vi "read_node_object_dictionary.vi"(0 "node":u8, 5 "index":u16, 7 "subind":u8, 9 "upd":u8, 11 "num":u64) -> (4 "return":i16, 6 "upd":u8, 8 "num":u64)   [LabVIEW 2011]
uses:
  canopen_dll_master.dll
panel:
  in  "num":cluster{"num":u64}
  in  "upd":cluster{"upd":u8}
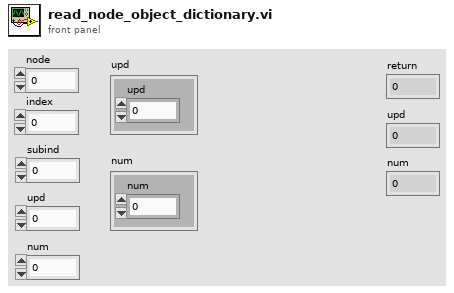
[diagram p1: front panel]
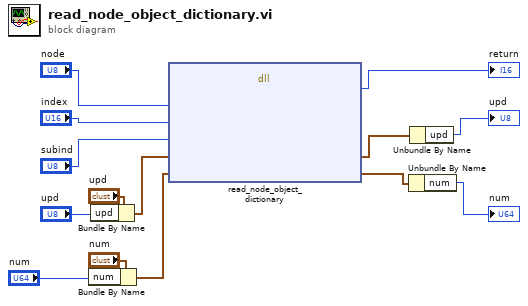
[diagram p0: block diagram]
diagram:
  n1 = Bundle By Name(cluster="num", "num"="num") -> (w3:cluster{"num":u64})
  n2 = Bundle By Name(cluster="upd", "upd"="upd") -> (w9:cluster{"upd":u8})
  n3 = dll-call lib="canopen_dll_master.dll" fn="read_node_object_dictionary"("node"="node", "index"="index", "subind"="subind", "upd"=w9, "num"=w3) -> ("return type"=→"return":i16, "upd"=w8:cluster{"upd":u8}, "num"=w2:cluster{"num":u64})  [unwired: 6 in, 2 out]
  n4 = Unbundle By Name(w2) -> ("num"=→"num":u64)
  n5 = Unbundle By Name(w8) -> ("upd"=→"upd":u8)
